vi "Draw_Calculate Height for Body.vi"(8 "Error":errorcluster, 11 "ICON Cluster":T1={"Header"="", "Body"=[], "ImageData"={"image type"=0, "image depth"=0, "image"=[], "mask"=[], "colors"=[], "Rectangle"={"left"=0, "top"=0, "right"=0, "bottom"=0}}, "New Icon"=bytes[0], "Line Status"=[], "Format"={"Color"={"Body txt"=255, "Body Back"=12632256, "Frame"=0, "Header txt"=32768, "Header Back"=16744703, "type"=enum."2 Color"}, "Icon Sizing"={"Rule"=enum."Static", "Header"=TRUE, "Rows"=5, "Width"=32, "Position"=enum."MID-CTR"}}} {"Format"."Icon Sizing"."Rows" min=1 max=5 step=1; "Format"."Icon Sizing"."Width" min=7 max=32 step=1}) -> (0 "Error Out":errorcluster, 3 "Height Out":u32)   [LabVIEW 2009]
uses:
  Controls/Cluster/Cluster_Icon Data.ctl
  Controls/String_Picture/STRING_Line Display.ctl
  Controls/Array/String Array_Body Text.ctl
  Controls/Cluster/Cluster_Image Data.ctl
  Controls/Cluster/CLuster_Selectoin Box.ctl
  Controls/String_Picture/Picture_Icon.ctl
  Controls/Cluster/Cluster_Icon Format.ctl
  Controls/Cluster/Cluster_Icon Color Set.ctl
  Controls/Enum/ENUM_Frame Template Select.ctl
  Controls/Cluster/Cluster_Sizing Data.ctl
  Controls/Enum/ENUM_Icon Sizing.ctl
  Controls/Enum/RBENUM_Icon Position.ctl
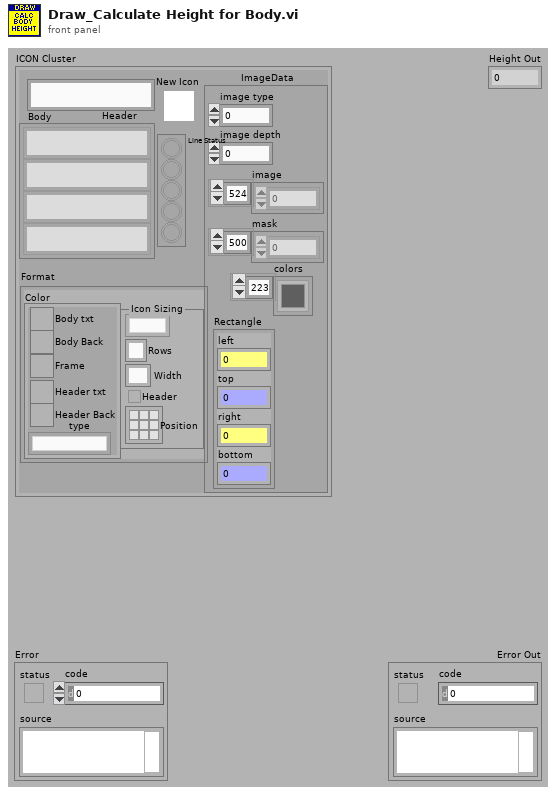
[diagram p1: front panel]
types:
  T1 = typedef "Cluster_Icon Data.ctl" = cluster{"Header":T2, "Body":T3, "ImageData":T4, "New Icon":T6, "Line Status":bool[], "Format":T7}
  T2 = typedef "STRING_Line Display.ctl" = string
  T3 = typedef "String Array_Body Text.ctl" = T2[]
  T4 = typedef "Cluster_Image Data.ctl" = cluster{"image type":i32, "image depth":i32, "image":u8[], "mask":u8[], "colors":u32[], "Rectangle":T5}
  T5 = typedef "CLuster_Selectoin Box.ctl" = cluster{"left":i16, "top":i16, "right":i16, "bottom":i16}
  T6 = typedef "Picture_Icon.ctl" = picture
  T7 = typedef "Cluster_Icon Format.ctl" = cluster{"Color":T8, "Icon Sizing":T10}
  T8 = typedef "Cluster_Icon Color Set.ctl" = cluster{"Body txt":u32, "Body Back":u32, "Frame":u32, "Header txt":u32, "Header Back":u32, "type":T9}
  T9 = typedef "ENUM_Frame Template Select.ctl" = enum16{"2 Color", "5 Color"}
  T10 = typedef "Cluster_Sizing Data.ctl" = cluster{"Rule":T11, "Header":bool, "Rows":u32, "Width":u32, "Position":T12}
  T11 = typedef "ENUM_Icon Sizing.ctl" = enum16{"Static", "Auto"}
  T12 = typedef "RBENUM_Icon Position.ctl" = enum32{"LFT-TOP", "MID-TOP", "RGT-TOP", "LFT-CTR", "MID-CTR", "RGT-CTR", "LFT-BOT", "MID-BOT", "RGT-BOT"}
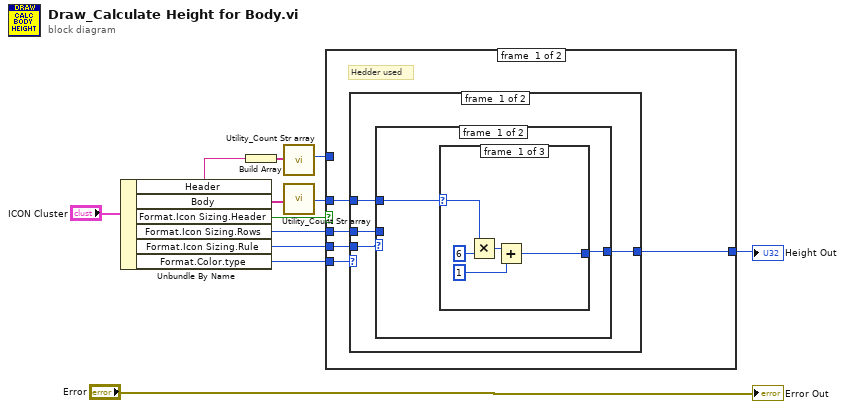
[diagram p0: block diagram]
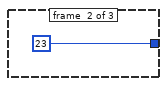
[diagram p2: hidden frame]
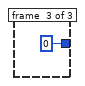
[diagram p3: hidden frame]
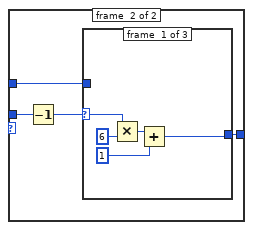
[diagram p4: hidden frame]
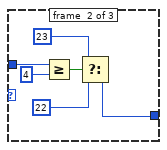
[diagram p5: hidden frame]
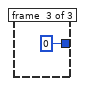
[diagram p6: hidden frame]
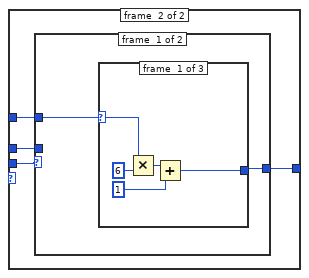
[diagram p7: hidden frame]
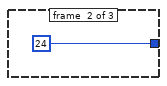
[diagram p8: hidden frame]
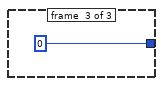
[diagram p9: hidden frame]
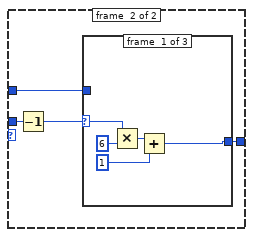
[diagram p10: hidden frame]
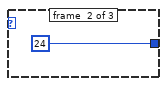
[diagram p11: hidden frame]
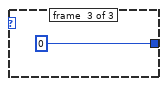
[diagram p12: hidden frame]
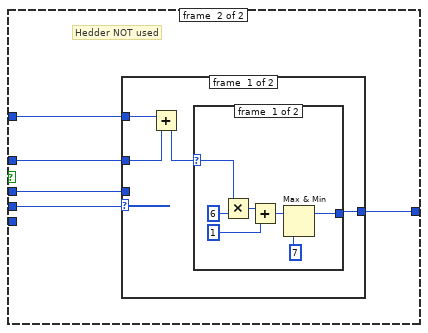
[diagram p13: hidden frame]
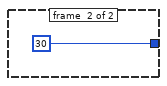
[diagram p14: hidden frame]
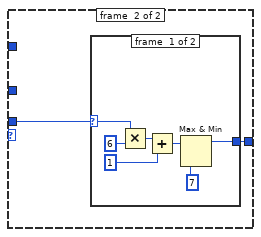
[diagram p15: hidden frame]
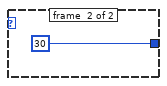
[diagram p16: hidden frame]
diagram:
  n1 = Unbundle By Name("ICON Cluster") -> ("Header"=w3:T2, "Body"=w5:T3, "Format.Icon Sizing.Header"=w9:bool, "Format.Icon Sizing.Rows"=w8:u32, "Format.Icon Sizing.Rule"=w7:T11, "Format.Color.type"=w6:T9)
  n2 = Build Array(w3) -> (w2:T2[])
  n3 = call "Utility_Count Str array.vi"("String Array"=w2) -> ("Count Out"=w1:i16)  [unwired: 8 in, 2 out]
  n4 = call "Utility_Count Str array.vi"("String Array"=w5) -> ("Count Out"=w4:i16)  [unwired: 8 in, 2 out]
  n5 = case shown="False" w9 {
    tunnel: [w17 w75] -> w10
    tunnel: w8 -> [w16 w74]
    tunnel: w4 -> [w14 w73]
    tunnel: w1 -> [_ w71]
    tunnel: w7 -> [w13 w72]
    tunnel: w6 -> [w15 _]
    frame #0 {
      # "Hedder used"
      n6 = case shown="\"2 Color\"" w15 {
        tunnel: [w21 w50] -> w17
        tunnel: w16 -> [w18 w47]
        tunnel: w14 -> [w20 w49]
        tunnel: w13 -> [w19 w48]
        frame #0 {
          n7 = case shown="\"Auto\"" w19 {
            tunnel: [w23 w34] -> w21
            tunnel: w20 -> [w22 w32]
            tunnel: w18 -> [_ w33]
            frame #0 {
              n8 = case shown="4.." w22 {
                selector: w22 -> [w28 _ _]
                tunnel: [w24 u32 23 u32 0] -> w23
                frame #0 {
                  n9 = Multiply(x=w28, y=u32 6) -> (x*y=w26:u32)
                  n10 = Add(x=w26, y=u32 1) -> (x+y=w24:u32)
                }
                frame #1 {
                }
                frame #2 {
                }
              }
            }
            frame #1 {
              n11 = Decrement(x=w33) -> (x-1=w31:u32)
              n12 = case shown="4.." w31 {
                selector: w31 -> [w39 _ _]
                tunnel: [w35 w40 u32 0] -> w34
                tunnel: w32 -> [_ w45 _]
                frame #0 {
                  n13 = Multiply(x=w39, y=u32 6) -> (x*y=w37:u32)
                  n14 = Add(x=w37, y=u32 1) -> (x+y=w35:u32)
                }
                frame #1 {
                  n15 = Greater Or Equal?(x=w45, y=4) -> (x >= y?=w43:bool)
                  n16 = Select(t=u32 23, s=w43, f=u32 22) -> (s? t:f=w40:u32)
                }
                frame #2 {
                }
              }
            }
          }
        }
        frame #1 {
          n17 = case shown="\"Auto\"" w48 {
            tunnel: [w52 w63] -> w50
            tunnel: w49 -> [w51 w61]
            tunnel: w47 -> [_ w62]
            frame #0 {
              n18 = case shown="4.." w51 {
                selector: w51 -> [w57 _ _]
                tunnel: [w53 u32 24 u32 0] -> w52
                frame #0 {
                  n19 = Multiply(x=w57, y=u32 6) -> (x*y=w55:u32)
                  n20 = Add(x=w55, y=u32 1) -> (x+y=w53:u32)
                }
                frame #1 {
                }
                frame #2 {
                }
              }
            }
            frame #1 {
              n21 = Decrement(x=w62) -> (x-1=w60:u32)
              n22 = case shown="4.." w60 {
                selector: w60 -> [w68 _ _]
                tunnel: [w64 u32 24 u32 0] -> w63
                tunnel: w61 -> [_ _ _]
                frame #0 {
                  n23 = Multiply(x=w68, y=u32 6) -> (x*y=w66:u32)
                  n24 = Add(x=w66, y=u32 1) -> (x+y=w64:u32)
                }
                frame #1 {
                }
                frame #2 {
                }
              }
            }
          }
        }
      }
    }
    frame #1 {
      # "Hedder NOT used"
      n25 = case shown="\"Auto\"" w72 {
        tunnel: [w79 w89] -> w75
        tunnel: w71 -> [w78 _]
        tunnel: w73 -> [w77 _]
        tunnel: w74 -> [_ w88]
        frame #0 {
          n26 = Add(x=w78, y=w77) -> (x+y=w76:i16)
          n27 = case shown="..4" w76 {
            selector: w76 -> [w86 _]
            tunnel: [w80 u32 30] -> w79
            frame #0 {
              n28 = Multiply(x=w86, y=u32 6) -> (x*y=w84:u32)
              n29 = Add(x=w84, y=u32 1) -> (x+y=w82:u32)
              n30 = Max & Min(x=w82, y=u32 7) -> (max(x,y)=w80:u32)  [unwired: 1 out]
            }
            frame #1 {
            }
          }
        }
        frame #1 {
          n31 = case shown="..4" w88 {
            selector: w88 -> [w96 _]
            tunnel: [w90 u32 30] -> w89
            frame #0 {
              n32 = Multiply(x=w96, y=u32 6) -> (x*y=w94:u32)
              n33 = Add(x=w94, y=u32 1) -> (x+y=w92:u32)
              n34 = Max & Min(x=w92, y=u32 7) -> (max(x,y)=w90:u32)  [unwired: 1 out]
            }
            frame #1 {
            }
          }
        }
      }
    }
  }
  "Height Out" <- w10
  "Error Out" <- "Error"
